vi "PhotonTrackedTarget_PopulatePacket.vi"(11 "TrackedTarget":T1={"Yaw"=0.0, "Pitch"=0.0, "Area"=0.0, "Skew"=0.0, "TargetCorners"=[], "CameraToTarget"={"TRANSLATION"={"X"=0.0, "Y"=0.0}, "ROTATION"={"VALUE"=0.0, "COS"=1.0, "SIN"=0.0}}} {"CameraToTarget"."ROTATION"."SIN" format="%13.4f"; "CameraToTarget"."ROTATION"."COS" format="%13.4f"; "CameraToTarget"."ROTATION"."VALUE" format="%13.4f"; "CameraToTarget"."TRANSLATION"."Y" format="%14.3f"; "CameraToTarget"."TRANSLATION"."X" format="%14.3f"}) -> (3 "RawData Out":u8[](array[numeric]))   [LabVIEW 2019, in "PhotonVisionLib.lvlib"]
doc: "Encode a TrackedTarget cluster into an array of bytes.\n\nInputs:\n - TrackedTarget -- TrackedTarget cluster.\n\nOutputs:\n - RawDataOut -- Byte array containing the encoded data."
uses:
  PhotonVisionLib.lvlib
  TypeDef/PhotonTrackedTargetType.ctl
  TypeDef/TargetCornerType.ctl
  <vilib>/Rock Robotics/WPI/ThirdParty/JAS_Junk/TrajLib/TRANSFORM2D.ctl
  <vilib>/Rock Robotics/WPI/ThirdParty/JAS_Junk/TrajLib/TRANSLATION2D.ctl
  <vilib>/Rock Robotics/WPI/ThirdParty/JAS_Junk/TrajLib/ROTATION2D.ctl
  <vilib>/Rock Robotics/WPI/ThirdParty/JAS_Junk/TrajLib/Trajectory_Library.lvlib
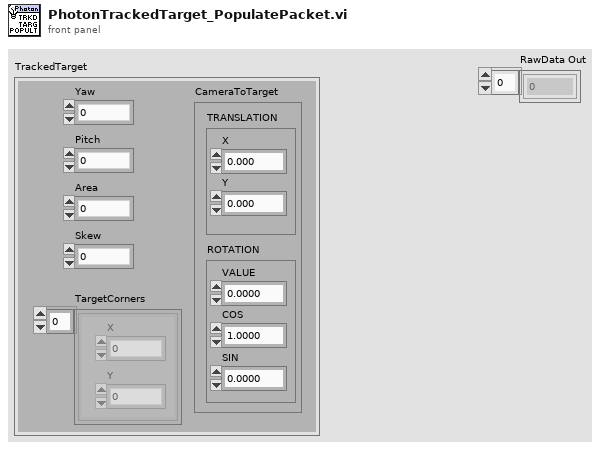
[diagram p1: front panel]
types:
  T1 = typedef "PhotonVisionLib.lvlib/PhotonTrackedTargetType.ctl" = cluster{"Yaw":dbl, "Pitch":dbl, "Area":dbl, "Skew":dbl, "TargetCorners":T2[], "CameraToTarget":T3}
  T2 = typedef "PhotonVisionLib.lvlib/TargetCornerType.ctl" = cluster{"X":dbl, "Y":dbl}
  T3 = typedef "Trajectory_Library.lvlib/TRANSFORM2D.ctl" = cluster{"TRANSLATION":T4, "ROTATION":T5}
  T4 = typedef "Trajectory_Library.lvlib/TRANSLATION2D.ctl" = cluster{"X":dbl, "Y":dbl}
  T5 = typedef "Trajectory_Library.lvlib/ROTATION2D.ctl" = cluster{"VALUE":dbl, "COS":dbl, "SIN":dbl}
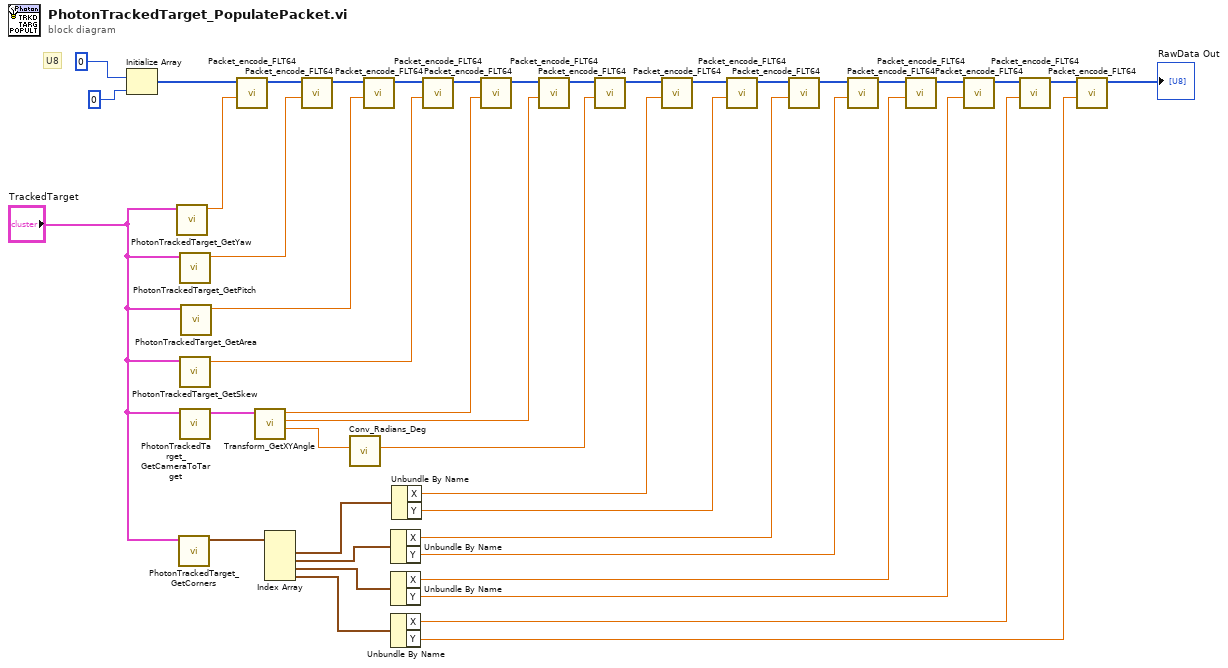
[diagram p0: block diagram]
diagram:
  # "U8"
  n1 = Initialize Array(u8 0 ("element"), 0 ("dimension size")) -> (w37:u8[])
  n2 = call "PhotonTrackedTarget_GetYaw.vi"("TrackedTarget"="TrackedTarget") -> ("Yaw"=w29:dbl)  [unwired: 10 in]
  n3 = call "PhotonTrackedTarget_GetCorners.vi"("TrackedTarget"="TrackedTarget") -> ("TargetCorners"=w22:T2[])  [unwired: 10 in]
  n4 = call "PhotonTrackedTarget_GetPitch.vi"("TrackedTarget"="TrackedTarget") -> ("Pitch"=w28:dbl)  [unwired: 10 in]
  n5 = call "PhotonTrackedTarget_GetSkew.vi"("TrackedTarget"="TrackedTarget") -> ("Skew"=w26:dbl)  [unwired: 10 in]
  n6 = call "PhotonTrackedTarget_GetCameraToTarget.vi"("TrackedTarget"="TrackedTarget") -> ("CameraToTarget"=w39:T3)  [unwired: 10 in]
  n7 = call "PhotonTrackedTarget_GetArea.vi"("TrackedTarget"="TrackedTarget") -> ("Area"=w27:dbl)  [unwired: 10 in]
  n8 = call "Packet_encode_FLT64.vi"("FLT64_Value"=w29, "RawData In"=w37) -> ("RawData Out"=w36:u8[])  [unwired: 9 in]
  n9 = call <vilib>:"Transform_GetXYAngle.vi"("inTRANSFORM"=w39) -> ("Angle"=w38:dbl, "Y"=w24:dbl, "X"=w25:dbl)  [unwired: 8 in]
  n10 = Index Array(array=w22) -> (element #1=w21:T2, element #2=w20:T2, element #3=w19:T2, element #4=w18:T2)  [unwired: 4 in]
  n11 = call "Packet_encode_FLT64.vi"("FLT64_Value"=w28, "RawData In"=w36) -> ("RawData Out"=w35:u8[])  [unwired: 9 in]
  n12 = call <vilib>:"Conv_Radians_Deg.vi"("Radians"=w38) -> ("Degrees"=w23:dbl)  [unwired: 10 in]
  n13 = call "Packet_encode_FLT64.vi"("FLT64_Value"=w27, "RawData In"=w35) -> ("RawData Out"=w34:u8[])  [unwired: 9 in]
  n14 = Unbundle By Name(w20) -> ("X"=w7:dbl, "Y"=w6:dbl)
  n15 = Unbundle By Name(w19) -> ("X"=w5:dbl, "Y"=w4:dbl)
  n16 = Unbundle By Name(w18) -> ("X"=w3:dbl, "Y"=w2:dbl)
  n17 = Unbundle By Name(w21) -> ("X"=w9:dbl, "Y"=w8:dbl)
  n18 = call "Packet_encode_FLT64.vi"("FLT64_Value"=w26, "RawData In"=w34) -> ("RawData Out"=w33:u8[])  [unwired: 9 in]
  n19 = call "Packet_encode_FLT64.vi"("FLT64_Value"=w25, "RawData In"=w33) -> ("RawData Out"=w32:u8[])  [unwired: 9 in]
  n20 = call "Packet_encode_FLT64.vi"("FLT64_Value"=w24, "RawData In"=w32) -> ("RawData Out"=w31:u8[])  [unwired: 9 in]
  n21 = call "Packet_encode_FLT64.vi"("FLT64_Value"=w23, "RawData In"=w31) -> ("RawData Out"=w11:u8[])  [unwired: 9 in]
  n22 = call "Packet_encode_FLT64.vi"("FLT64_Value"=w9, "RawData In"=w11) -> ("RawData Out"=w17:u8[])  [unwired: 9 in]
  n23 = call "Packet_encode_FLT64.vi"("FLT64_Value"=w8, "RawData In"=w17) -> ("RawData Out"=w16:u8[])  [unwired: 9 in]
  n24 = call "Packet_encode_FLT64.vi"("FLT64_Value"=w7, "RawData In"=w16) -> ("RawData Out"=w15:u8[])  [unwired: 9 in]
  n25 = call "Packet_encode_FLT64.vi"("FLT64_Value"=w6, "RawData In"=w15) -> ("RawData Out"=w14:u8[])  [unwired: 9 in]
  n26 = call "Packet_encode_FLT64.vi"("FLT64_Value"=w5, "RawData In"=w14) -> ("RawData Out"=w13:u8[])  [unwired: 9 in]
  n27 = call "Packet_encode_FLT64.vi"("FLT64_Value"=w4, "RawData In"=w13) -> ("RawData Out"=w12:u8[])  [unwired: 9 in]
  n28 = call "Packet_encode_FLT64.vi"("FLT64_Value"=w3, "RawData In"=w12) -> ("RawData Out"=w10:u8[])  [unwired: 9 in]
  n29 = call "Packet_encode_FLT64.vi"("FLT64_Value"=w2, "RawData In"=w10) -> ("RawData Out"=→"RawData Out":u8[])  [unwired: 9 in]
